vi "dpu_cfg_read.vi"(8 "error in":errorcluster, 11 "master":refnum<class "Modbus Master.lvclass">) -> (0 "error out":errorcluster, 2 "DPU_CFG":T1 {"CAL_DATE" format="%08d"}, 3 "master":refnum<class "Modbus Master.lvclass">)   [LabVIEW 2014]
uses:
  protocol/modbus/ni_modbus_api/API/Master/Modbus Master.lvclass
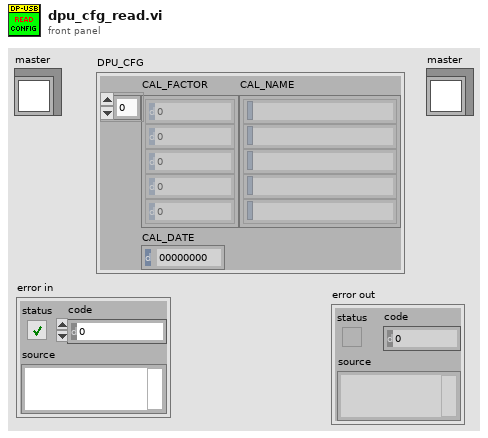
[diagram p1: front panel]
types:
  T1 = cluster{"CAL_FACTOR":sgl[], "CAL_DATE":u32, "CAL_NAME":string[]}
  T2 = enum16{"big-endian, network order", "native, host order", "little-endian"}
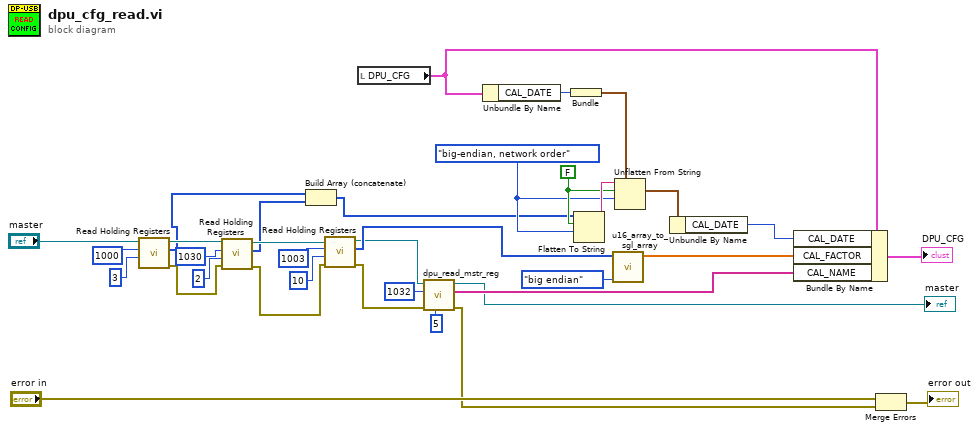
[diagram p0: block diagram]
diagram:
  w22 = T2."big-endian, network order" ("byte order (0:big-endian, network order)")
  w23 = FALSE ("prepend array or string size? (T)")
  n1 = call-dynamic "Read Holding Registers.vi"("number of inputs"=u16 3 ("Quantity"), "starting address"=u16 1000 ("Starting Address"), "Modbus master in"="master") -> ("error out"=w15:errorcluster, "register values"=w18:u16[], "Modbus master out"=w20:refnum<class "Modbus Master.lvclass">)  [unwired: 6 in]
  n2 = call-dynamic "Read Holding Registers.vi"("error in"=w15, "number of inputs"=u16 2 ("Quantity"), "starting address"=u16 1030 ("Starting Address"), "Modbus master in"=w20) -> ("error out"=w14:errorcluster, "register values"=w17:u16[], "Modbus master out"=w19:refnum<class "Modbus Master.lvclass">)  [unwired: 5 in]
  n3 = Build Array (concatenate)(w18, w17) -> (w13:u16[])
  n4 = call-dynamic "Read Holding Registers.vi"("error in"=w14, "number of inputs"=u16 10 ("Quantity"), "starting address"=u16 1003 ("Starting Address"), "Modbus master in"=w19) -> ("error out"=w9:errorcluster, "register values"=w5:u16[], "Modbus master out"=w4:refnum<class "Modbus Master.lvclass">)  [unwired: 5 in]
  n5 = local read "DPU_CFG"() -> (w28:T1)
  n6 = call "dpu_read_mstr_reg.vi"("num of str"=5, "error in"=w9, "first str reg"=u16 1032, "master"=w4) -> ("error out"=w1:errorcluster, "strings"=w6:string[], "master out"=→"master":refnum<class "Modbus Master.lvclass">)  [unwired: 4 in, 1 out]
  n7 = Unbundle By Name(w28) -> ("CAL_DATE"=w12:u32)
  n8 = Bundle("CAL_DATE"=w12) -> (w30:cluster{"CAL_DATE":u32})  [unwired: 1 in]
  n9 = Flatten To String(anything=w13, prepend array or string size? (T)=w23, byte order (0:big-endian, network order)=w22) -> (data string=w31:string)  [unwired: 1 in, 2 out]
  n10 = call "u16_array_to_sgl_array.vi"("word order"=enum16{"little endian", "big endian"}."big endian", "Regs_u16"=w5) -> ("VAL_sgl"=w11:sgl[])  [unwired: 9 in]
  n11 = Unflatten From String(type=w30, binary string=w31, data includes array or string size? (T)=w23, byte order (0:big-endian, network order)=w22) -> (value=w29:cluster{"CAL_DATE":u32})  [unwired: 1 in, 2 out]
  n12 = Unbundle By Name(w29) -> ("CAL_DATE"=w10:u32)
  n13 = Bundle By Name(cluster=w28, "CAL_DATE"=w10, "CAL_FACTOR"=w11, "CAL_NAME"=w6) -> (→"DPU_CFG":T1)
  n14 = Merge Errors("error in", w1) -> (→"error out":errorcluster)
